vi "PH_Beckhoff_Application.declare Tags.vi"(2 "error in":errorcluster, 3 "Instance Name":string) -> (0 "error out":errorcluster, 1 "Data in cluster":T1={"Default Values"={"Sonderklemmen Inputs"=[], "Analog Inputs"=[], "Analog Outputs"=[], "Digital Inputs"=[], "Digital Outputs"=[]}, "Description"="", "Hardware configured?"=TRUE, "Activate Change Manager?"=FALSE, "Difference to handle an analog input as change"=1})   [LabVIEW 2014, in "PH_Beckhoff_Application.lvlib"]
doc: "This VI declares the tagnames and sets the scaling of the tags of this class."
uses:
  PH_Beckhoff_Application.lvlib
  PH_Beckhoff/PH_Beckhoff.constructor Data in.ctl
  PH_Beckhoff/PH_Beckhoff.Values.ctl
  PH_Beckhoff/PH_Beckhoff.Sonderklemmen Inputs.ctl
  PH_Beckhoff/PH_Beckhoff.Analog Inputs.ctl
  PH_Beckhoff/PH_Beckhoff.Scaling Type.ctl
  PH_Beckhoff/PH_Beckhoff.Analog Outputs.ctl
  PH_Beckhoff/PH_Beckhoff.Digital Inputs.ctl
  PH_Beckhoff/PH_Beckhoff.Digital Outputs.ctl
  PH_Beckhoff/PH_Beckhoff.lvlib
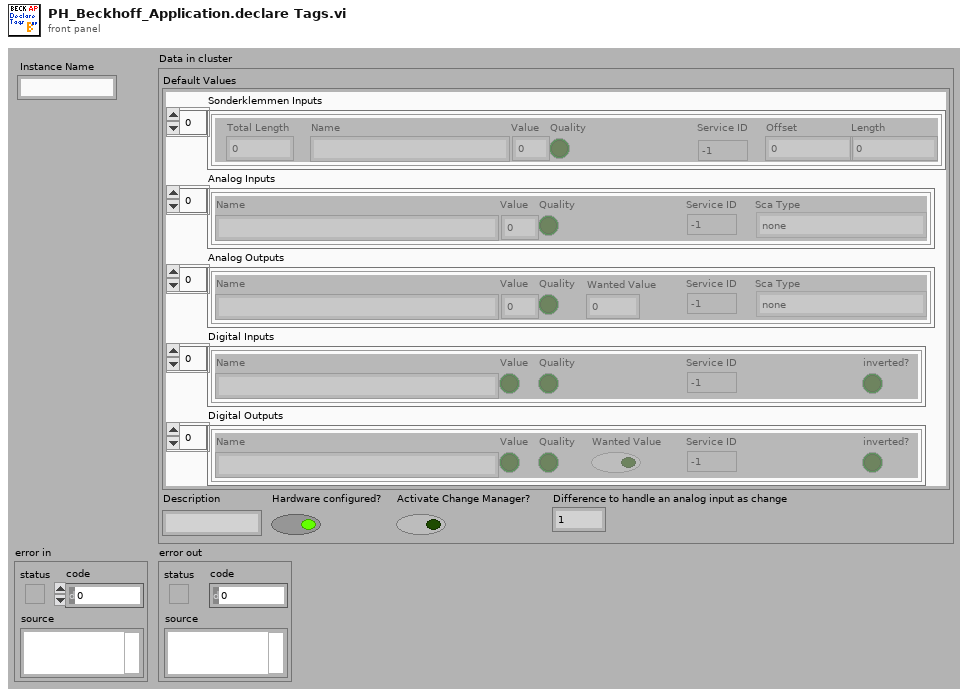
[diagram p1: front panel]
types:
  T1 = typedef "PH_Beckhoff.lvlib/PH_Beckhoff.constructor Data in.ctl" = cluster{"Default Values":T2, "Description":string, "Hardware configured?":bool, "Activate Change Manager?":bool, "Difference to handle an analog input as change":u32}
  T2 = typedef "PH_Beckhoff.lvlib/PH_Beckhoff.Values.ctl" = cluster{"Sonderklemmen Inputs":T3, "Analog Inputs":T4, "Analog Outputs":T6, "Digital Inputs":T7, "Digital Outputs":T8}
  T3 = typedef "PH_Beckhoff.lvlib/PH_Beckhoff.Sonderklemmen Inputs.ctl" = cluster{"Total Length":u32, "Name":string, "Value":u64, "Quality":bool, "Service ID":i32, "Offset":u32, "Length":u32}[]
  T4 = typedef "PH_Beckhoff.lvlib/PH_Beckhoff.Analog Inputs.ctl" = cluster{"Name":string, "Value":u32, "Quality":bool, "Service ID":i32, "Sca Type":T5}[]
  T5 = typedef "PH_Beckhoff.lvlib/PH_Beckhoff.Scaling Type.ctl" = enum16{"none", "0 ... 15 Bit -> 0 ... 5", "0 ... 15 Bit -> 0 ... 10", "0 ... 15 Bit -> 0 ... 25", "0 ... 15 Bit -> 4 ... 20", "0 ... 15 Bit -> 0 ... 1", "0 ... 15 Bit -> 0 ... 20000", "0 ... 15 Bit -> 0 ... 24000"}
  T6 = typedef "PH_Beckhoff.lvlib/PH_Beckhoff.Analog Outputs.ctl" = cluster{"Name":string, "Value":u32, "Quality":bool, "Wanted Value":u32, "Service ID":i32, "Sca Type":T5}[]
  T7 = typedef "PH_Beckhoff.lvlib/PH_Beckhoff.Digital Inputs.ctl" = cluster{"Name":string, "Value":bool, "Quality":bool, "Service ID":i32, "inverted?":bool}[]
  T8 = typedef "PH_Beckhoff.lvlib/PH_Beckhoff.Digital Outputs.ctl" = cluster{"Name":string, "Value":bool, "Quality":bool, "Wanted Value":bool, "Service ID":i32, "inverted?":bool}[]
  T9 = typedef "PH_Beckhoff_Application.lvlib/PH_Beckhoff_Application.Beckhoff Type.ctl" = enum16{"none", "PILS internal", "PILS external", "Timing", "MA 01"}
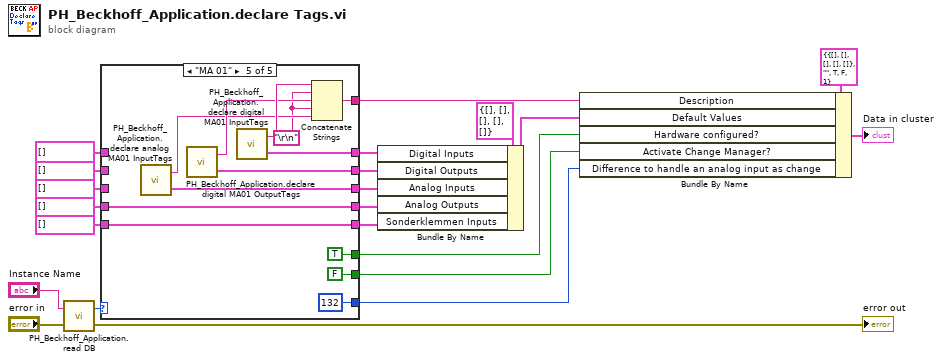
[diagram p0: block diagram]
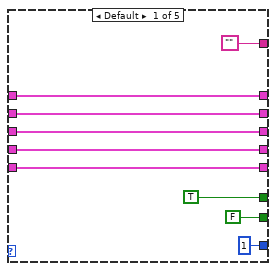
[diagram p2: hidden frame]
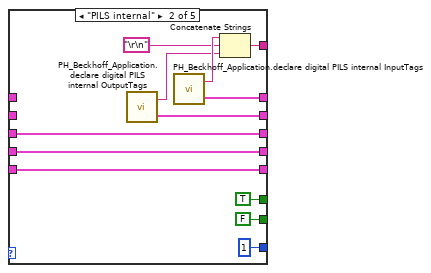
[diagram p3: hidden frame]
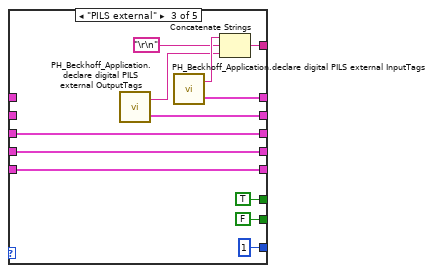
[diagram p4: hidden frame]
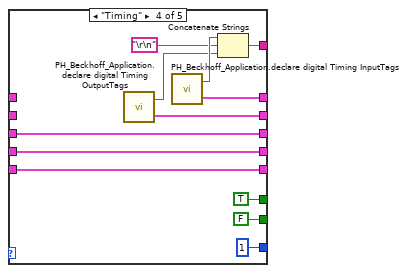
[diagram p5: hidden frame]
diagram:
  n1 = call "PH_Beckhoff_Application.read DB.vi"("error in"="error in", "Instance Name"="Instance Name") -> ("error out"=→"error out":errorcluster, "Beckhoff Type"=w6:T9)
  n2 = case shown="\"MA 01\"" w6 {
    tunnel: [w25 w32 w44 w58 w74] -> w19
    tunnel: [w26 w33 w45 w57 w68] -> w15
    tunnel: ["" w41 w53 w65 w78] -> w13
    tunnel: [w27 w34 w46 w56 w69] -> w12
    tunnel: [w24 w39 w51 w63 w77] -> w11
    tunnel: [w23 w38 w50 w62 w76] -> w10
    tunnel: [TRUE ("Hardware configured?") TRUE ("Hardware configured?") TRUE ("Hardware configured?") TRUE ("Hardware configured?") TRUE ("Hardware configured?")] -> w9
    tunnel: [FALSE FALSE FALSE FALSE FALSE] -> w8
    tunnel: [u32 1 ("Difference to handle an analog input as change") u32 1 ("Difference to handle an analog input as change") u32 1 ("Difference to handle an analog input as change") u32 1 ("Difference to handle an analog input as change") u32 132 ("Difference to handle an analog input as change")] -> w7
    tunnel: T3 [] ("Sonderklemmen Inputs") -> [w27 w34 w46 w56 w69]
    tunnel: T6 [] ("Analog Outputs") -> [w26 w33 w45 w57 w68]
    tunnel: T4 [] ("Analog Inputs") -> [w25 w32 w44 w58 _]
    tunnel: T8 [] ("Digital Outputs") -> [w24 _ _ _ _]
    tunnel: T7 [] ("Digital Inputs") -> [w23 _ _ _ _]
    frame Default {
    }
    frame "PILS internal" {
      n3 = call "PH_Beckhoff_Application.declare digital PILS internal OutputTags.vi"() -> ("Digital Outputs"=w39:T8, "Description"=w42:string)  [unwired: 2 in]
      n4 = call "PH_Beckhoff_Application.declare digital PILS internal InputTags.vi"() -> ("Digital Inputs"=w38:T7, "Description"=w43:string)  [unwired: 2 in]
      n5 = Concatenate Strings(w43, "\r\n", w42) -> (w41:string)
    }
    frame "PILS external" {
      n6 = call "PH_Beckhoff_Application.declare digital PILS external OutputTags.vi"() -> ("Digital Outputs"=w51:T8, "Description"=w54:string)  [unwired: 2 in]
      n7 = call "PH_Beckhoff_Application.declare digital PILS external InputTags.vi"() -> ("Digital Inputs"=w50:T7, "Description"=w55:string)  [unwired: 2 in]
      n8 = Concatenate Strings(w55, "\r\n", w54) -> (w53:string)
    }
    frame "Timing" {
      n9 = call "PH_Beckhoff_Application.declare digital Timing OutputTags.vi"() -> ("Digital Outputs"=w63:T8, "Description"=w66:string)  [unwired: 2 in]
      n10 = call "PH_Beckhoff_Application.declare digital Timing InputTags.vi"() -> ("Digital Inputs"=w62:T7, "Description"=w67:string)  [unwired: 2 in]
      n11 = Concatenate Strings(w67, "\r\n", w66) -> (w65:string)
    }
    frame "MA 01" {
      w72 = "\r\n"
      n12 = call "PH_Beckhoff_Application.declare analog MA01 InputTags.vi"() -> ("Analog Inputs"=w74:T4, "Description"=w73:string)
      n13 = call "PH_Beckhoff_Application.declare digital MA01 OutputTags.vi"() -> ("Digital Outputs"=w77:T8, "Description"=w79:string)
      n14 = call "PH_Beckhoff_Application.declare digital MA01 InputTags.vi"() -> ("Digital Inputs"=w76:T7, "Description"=w80:string)
      n15 = Concatenate Strings(w80, w72, w79, w72, w73) -> (w78:string)
    }
  }
  n16 = Bundle By Name(cluster=T2 {"Sonderklemmen Inputs"=[], "Analog Inputs"=[], "Analog Outputs"=[], "Digital Inputs"=[], "Digital Outputs"=[]} ("Dummy Default Values"), "Digital Inputs"=w10, "Digital Outputs"=w11, "Analog Inputs"=w19, "Analog Outputs"=w15, "Sonderklemmen Inputs"=w12) -> (w16:T2)
  n17 = Bundle By Name(cluster=T1 {"Default Values"={"Sonderklemmen Inputs"=[], "Analog Inputs"=[], "Analog Outputs"=[], "Digital Inputs"=[], "Digital Outputs"=[]}, "Description"="", "Hardware configured?"=TRUE, "Activate Change Manager?"=FALSE, "Difference to handle an analog input as change"=1} ("Dummy data in cluster"), "Description"=w13, "Default Values"=w16, "Hardware configured?"=w9, "Activate Change Manager?"=w8, "Difference to handle an analog input as change"=w7) -> (→"Data in cluster":T1)
